vi "WritExcelValues.vi"(0 "Worksheets":refnum<k7>, 5 "表单Index":i32=1 min=1 step=1, 7 "位置":string[](array[string]), 9 "数据":string[](array[string]), 11 "error out":errorcluster) -> (15 "error out 2":errorcluster caption="error out")   [LabVIEW 2017]
panel:
  in  "Excel._Application 2":refnum<k7>
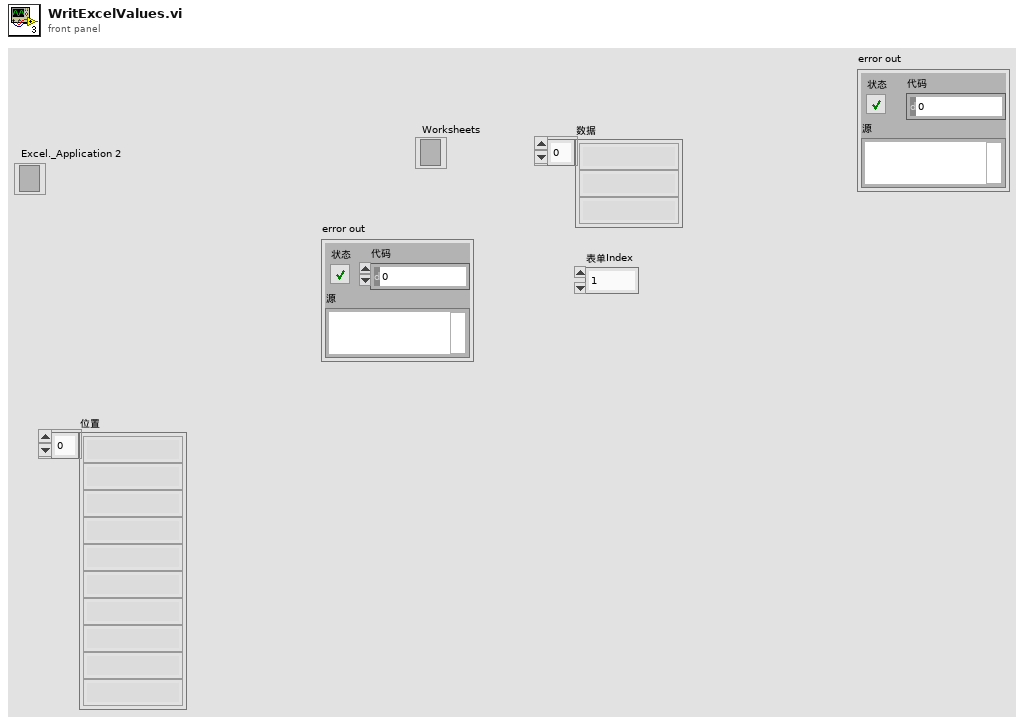
[diagram p1: front panel]
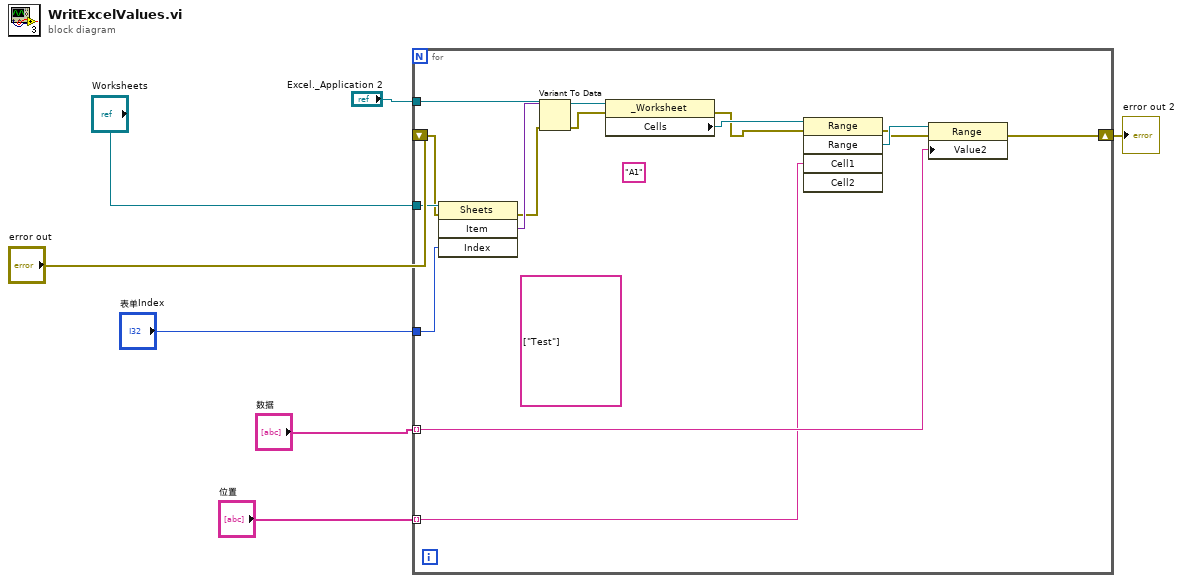
[diagram p0: block diagram]
diagram:
  n1 = for {
    tunnel: "Worksheets" -> [w22]
    tunnel: "Excel._Application 2" -> [w20]
    tunnel: "数据" -> [w12] mode=indexing
    shift-right: [w13] -> w3
    shift-left: "error out" -> [w17]
    tunnel: "表单Index" -> [w11]
    tunnel: "位置" -> [w10] mode=indexing
    (unwired) string[] ["Test"]
    (unwired) "A1"
    n2 = invoke on="调用节点" class="Sheets" method="Item"(reference=w22, error in=w17, "Index"=w11) -> (error out=w16:errorcluster, "Item"=w21:variant)  [unwired: 1 in, 2 out]
    n3 = Variant To Data(error in=w16, type=w20, Variant=w21) -> (data=w19:refnum<k7>, error out=w15:errorcluster)
    n4 = property on="属性节点" class="_Worksheet"(reference=w19, error in=w15) -> (error out=w14:errorcluster, "Cells"=w18:refnum<k7>)  [unwired: 1 out]
    n5 = invoke on="调用节点" class="Range" method="Range"(reference=w18, error in=w14, "Cell1"=w10) -> (error out=w8:errorcluster, "Range"=w9:refnum<k7>)  [unwired: 2 in, 3 out]
    n6 = property on="属性节点" class="Range"(reference=w9, error in=w8, "Value2"=w12) -> (error out=w13:errorcluster)  [unwired: 1 out]
  }
  "error out 2" <- w3
